vi "Update Step Time Remaining.vi"(8 "error in (no error)":errorcluster, 10 "Current Time":timestamp, 11 "Output Sequencer in":refnum<class "Output Sequencer.lvclass">) -> (0 "error out":errorcluster, 3 "Output Sequencer out":refnum<class "Output Sequencer.lvclass">)   [LabVIEW 2020, in "Output Sequencer.lvlib" / "Output Sequencer.lvclass"]
uses:
  Output Sequencer.lvclass
  Output Sequencer.lvclass/Output Sequencer.ctl
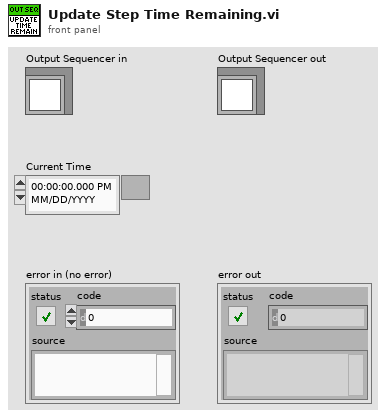
[diagram p1: front panel]
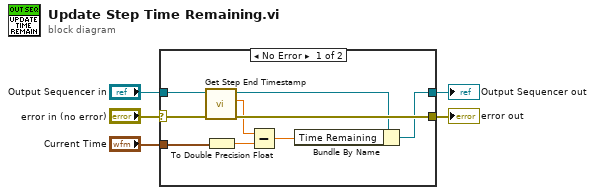
[diagram p0: block diagram]
diagram:
  n1 = case shown="No Error" "error in (no error)" {
    selector: "error in (no error)" -> [w6 w16]
    tunnel: [w14 w16] -> w5
    tunnel: [w13 w15] -> w4
    tunnel: "Current Time" -> [w12 _]
    tunnel: "Output Sequencer in" -> [w11 w15]
    frame No Error {
      n2 = call "Get Step End Timestamp.vi"("error in (no error)"=w6, "Output Sequencer in"=w11) -> ("error out"=w14:errorcluster, "Current Step End Timestamp"=w10:dbl, "Output Sequencer out"=w7:refnum<class "Output Sequencer.lvclass">)  [unwired: 7 in]
      n3 = To Double Precision Float(number=w12) -> (double precision float=w9:dbl)
      n4 = Subtract(x=w10, y=w9) -> (x-y=w8:dbl)
      n5 = Bundle By Name(cluster=w7, "Time Remaining"=w8) -> (w13:refnum<class "Output Sequencer.lvclass">)
    }
    frame Error {
    }
  }
  "error out" <- w5
  "Output Sequencer out" <- w4
